vi "Format Tree.vi"(8 "error in (no error)":errorcluster, 10 "Tag":string, 11 "Test Executive View in":refnum<class "Test Executive View.lvclass">) -> (0 "error out":errorcluster, 3 "Test Executive View out":refnum<class "Test Executive View.lvclass">)   [LabVIEW 2017, in "Test Executive View.lvclass"]
uses:
  <vilib>/gpm_packages/@cs/Test-executive-builder/Example/Application/Test Executive View/Test Executive View/Test Executive View.lvclass
  <vilib>/gpm_packages/@cs/Test-executive-builder/Source/Test Executive Builder View/Test Executive Builder View/Test Executive Builder View.lvclass
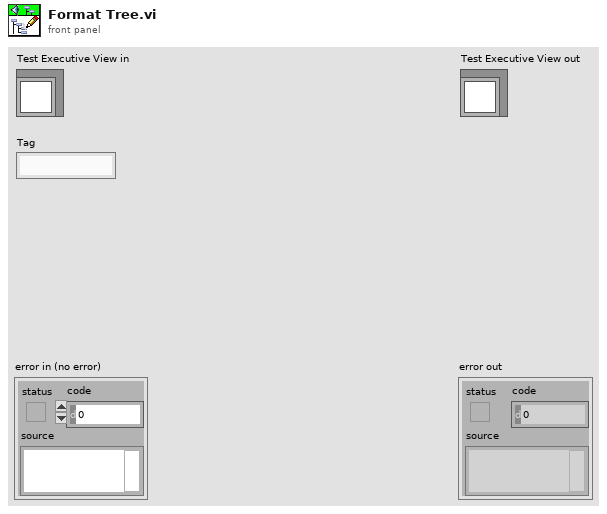
[diagram p1: front panel]
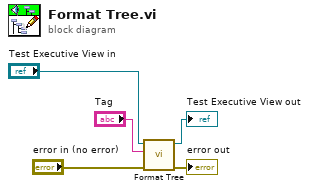
[diagram p0: block diagram]
diagram:
  n1 = call-parent "Format Tree.vi"("error in (no error)"="error in (no error)", "Tag"="Tag", "Test Executive Builder View in"="Test Executive View in") -> ("error out"=→"error out":errorcluster, "Test Executive Builder View out"=→"Test Executive View out":refnum<class "Test Executive View.lvclass">)  [unwired: 7 in]
